vi "testttt_Init.vi"(8 "ErrorIn":errorcluster caption="Error In", 11 "ObjectIn":refnum<class "testttt.lvclass"> caption="Object In") -> (0 "ErrorOut":errorcluster caption="Error Out", 3 "ObjectOut":refnum<class "testttt.lvclass"> caption="Object Out")   [LabVIEW 2018, in "testttt.lvclass"]
uses:
  <userlib>/_express/CustomErrorCreator/ErrorDefinitionSQLite/testttt/testttt.lvclass
  <userlib>/_express/CustomErrorCreator/ErrorDefinitionSQLite/testttt/testttt.lvclass/testttt.ctl
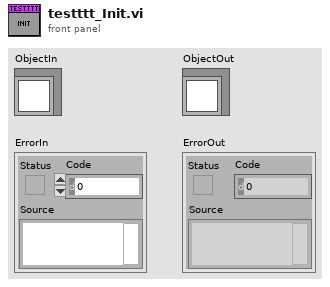
[diagram p1: front panel]
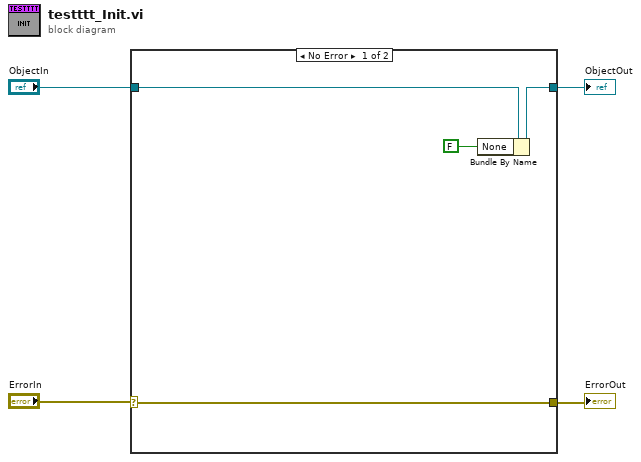
[diagram p0: block diagram]
diagram:
  n1 = case shown="No Error" "ErrorIn" {
    selector: "ErrorIn" -> [w5 w9]
    tunnel: "ObjectIn" -> [w6 w10]
    tunnel: [w8 w10] -> w3
    tunnel: [w5 w9] -> w1
    frame No Error {
      n2 = Bundle By Name(cluster=w6, "None"=FALSE) -> (w8:refnum<class "testttt.lvclass">)
    }
    frame Error {
    }
  }
  "ObjectOut" <- w3
  "ErrorOut" <- w1
